vi "MD5 (String).vi"(10 "message":string) -> (2 "MD5 hash":string)   [LabVIEW 2013, in "MD5.lvlib"]
uses:
  MD5.lvlib
  MD5.lvclass
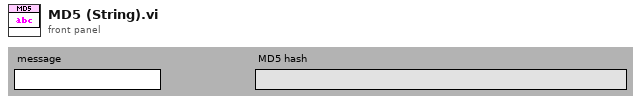
[diagram p1: front panel]
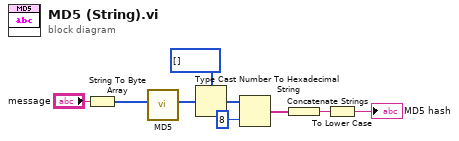
[diagram p0: block diagram]
diagram:
  n1 = String To Byte Array(string="message") -> (unsigned byte array=w8:u8[])
  n2 = call "MD5.vi"("data"=w8) -> ("MD5 hash"=w2:u8[])  [unwired: 10 in]
  n3 = Type Cast(type=u32[] [] ("U32"), x=w2) -> (*(type *) &x=w5:u32[])
  n4 = Number To Hexadecimal String(1:i16 8 ("width (-)"), 2:w5) -> (0:w4:string[])
  n5 = Concatenate Strings(w4) -> (w3:string)
  n6 = To Lower Case(string=w3) -> (all lower case string=→"MD5 hash":string)
